vi "estruturas_dados_cluster.vi"() -> ()   [LabVIEW 2013]
panel:
  in  "Enum":T1(ring)
  in  "stop":bool
  out "Aprovado":bool
  out "Nome":string
  out "Cod":dbl
  in  "App Cluster":T2
  # "Criação de controles e indicadores de cluster"
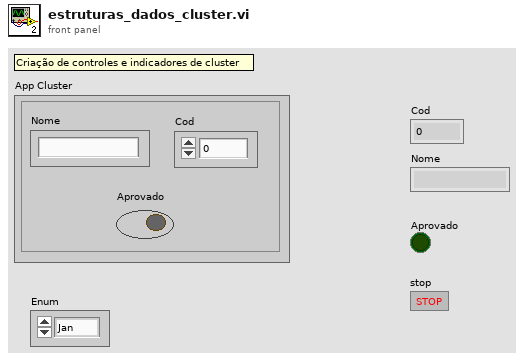
[diagram p1: front panel]
types:
  T1 = enum16{"Jan", "Fev", "Mar", "Abr", "Mai", "Jun", "Jul"}
  T2 = cluster{"Cod":dbl, "Nome":string, "Aprovado":bool}
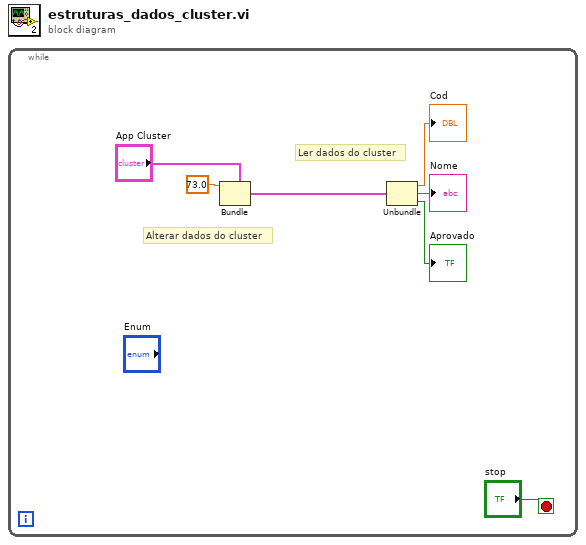
[diagram p0: block diagram]
diagram:
  n1 = while {
    stop <- "stop" stop-if-true
    # "Alterar dados do cluster"
    # "Ler dados do cluster"
    n2 = Bundle(cluster="App Cluster", "Cod"=73.0) -> (w1:T2)  [unwired: 2 in]
    n3 = Unbundle(w1) -> ("Cod"=→"Cod":dbl, "Nome"=→"Nome":string, "Aprovado"=→"Aprovado":bool)
  }
